vi "LVClass_Image data subtraction ABC.vi"(0 "Image C result":refnum<class "Image.lvclass">, 5 "image A":refnum<class "Image.lvclass">, 7 "image B to remove":refnum<class "Image.lvclass">, 11 "error in (no error)":errorcluster) -> (4 "Image out":refnum<class "Image.lvclass">, 15 "error out":errorcluster)   [LabVIEW 2020, in "Image.lvclass"]
doc: "Subtraction : Image = ImageA \\- ImageB. Images must have the same size,\nchannels count and bits depth.\n\n--------------------------------------------------------------------------------\n\n<B>ImageAIn </B> : Image object.\n<B>ImageAOut </B> : Image object.\n<B>ImageB </B> : Image object.\n<B>Image </B> : Image object.\n<B>ErrorIn </B> : Error\n<B>ErrorOut </B> : Error\n\n--------------------------------------------------------------------------------"
uses:
  Image.lvclass
  LVClass_Image read Image Compat ptr.vi
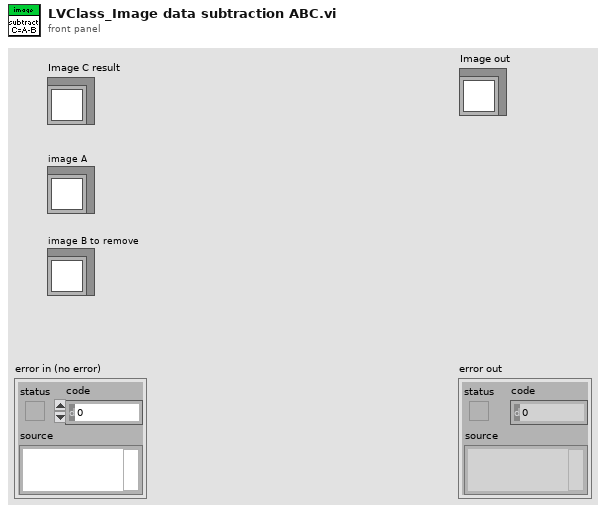
[diagram p1: front panel]
types:
  T1 = typedef "ClassID.ctl" = i64
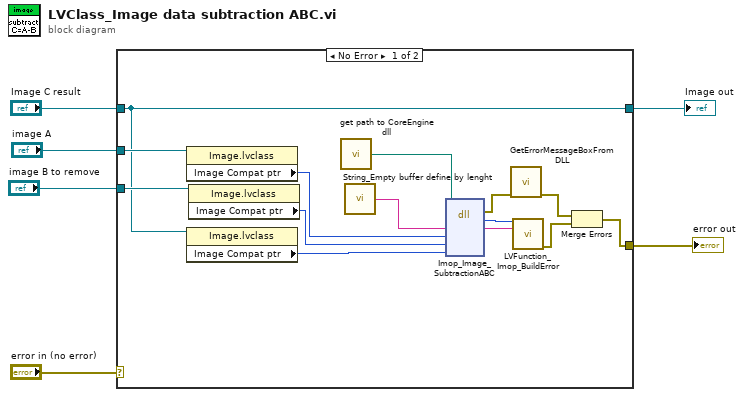
[diagram p0: block diagram]
diagram:
  n1 = case shown="No Error" "error in (no error)" {
    selector: "error in (no error)" -> [_ w22]
    tunnel: [w7 w22] -> w5
    tunnel: [w11 w21] -> w3
    tunnel: "Image C result" -> [w11 w21]
    tunnel: "image A" -> [w17 _]
    tunnel: "image B to remove" -> [w14 _]
    frame No Error {
      n2 = property class="Image.lvclass"(reference=w17) -> ("Image Compat ptr"=w13:T1)  [unwired: 1 in, 2 out]
      n3 = property class="Image.lvclass"(reference=w11) -> ("Image Compat ptr"=w10:T1)  [unwired: 1 in, 2 out]
      n4 = property class="Image.lvclass"(reference=w14) -> ("Image Compat ptr"=w12:T1)  [unwired: 1 in, 2 out]
      n5 = call "get path to CoreEngine dll.vi"() -> ("path to wavekit library"=w16:path)  [unwired: 14 in, 1 out]
      n6 = call "String_Empty buffer define by lenght.vi"() -> ("Empty buffer"=w20:string)  [unwired: 1 in]
      n7 = dll-call lib="D:/2_trunk/Soft_haso/ImOpCoreEngine4_LV2011/DLLs/ImopEngine4_vc100.dll" fn="Imop_Image_SubtractionABC"(path in=w16, "message"=w20, "Image 1"=w13, "Image 2"=w12, "Image3"=w10) -> (error out=w15:errorcluster, "return type"=w19:i32, "message"=w18:string)  [unwired: 5 in, 1 out]
      n8 = call "GetErrorMessageBoxFromDLL.vi"("error IN"=w15) -> ("error OUT"=w9:errorcluster)  [unwired: 10 in]
      n9 = call "LVFunction_Imop_BuildError.vi"("code"=w19, "String to Prepend to source (\"\")"=w18) -> ("error out"=w8:errorcluster)  [unwired: 13 in]
      n10 = Merge Errors(w9, w8) -> (w7:errorcluster)
    }
    frame Error {
    }
  }
  "error out" <- w5
  "Image out" <- w3
